vi "Load State Machine.vi"(11 "Autonomous? (Default false)":bool) -> (3 "Done (For Auto Use Only)":bool)   [LabVIEW 2013]
uses:
  typedefs/singleUseSubstate.ctl
  typedefs/fg_typedef.ctl
  typedefs/DevRef Type.ctl
  <vilib>/Rock Robotics/WPI/Solenoid/WPI_SolenoidValue.ctl
  typedefs/subStates.ctl
  <vilib>/Rock Robotics/WPI/Solenoid/WPI_SolenoidGetEnum.vi
panel:
  # "A State Machine to Handle Loading for Either High or Low Goal Shots"
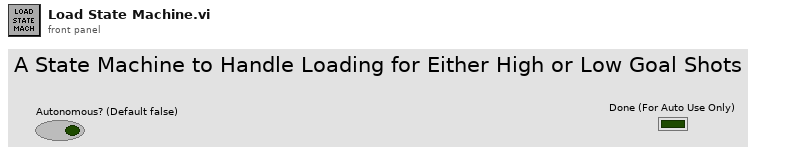
[diagram p1: front panel]
types:
  T1 = typedef "WPI_SolenoidValue.ctl" = enum16{"Off", "On", "Forward", "Reverse"}
  T2 = typedef "DevRef Type.ctl" = enum16{"Shooter Solenoid", "Latch Solenoid", "Right Up Sensor", "Right Down Sensor", "Hold Sensor", "Arm Encoder"}
  T3 = typedef "fg_typedef.ctl" = enum16{"Get", "Set"}
  T4 = typedef "singleUseSubstate.ctl" = enum16{"null", "wait", "shift high", "shift low", "extend shooter", "retract shooter", "latch", "unlatch"}
  T5 = typedef "subStates.ctl" = enum16{"null", "wait", "driver control", "auto", "manual override", "hold position", "rotate", "pickup", "pass", "load", "goto shoot", "shoot high goal", "shoot low goal", "cancel arm", "cancel shooter", "end"}
  T6 = typedef "WPI_SolenoidDevRef.ctl" = cluster{"DevStatus":errorcluster, "Solenoid Module":T7, "Forward Solenoid Channel":T8, "Reverse Solenoid Channel":T8}
  T7 = typedef "FPGA_TypedefSolenoidModule.ctl" = enum16{"Solenoid Module 1", "Solenoid Module 2"}
  T8 = typedef "WPI_SolenoidChannel.ctl" = enum8{"Solenoid 1", "Solenoid 2", "Solenoid 3", "Solenoid 4", "Solenoid 5", "Solenoid 6", "Solenoid 7", "Solenoid 8", "Invalid"}
  T9 = typedef "WPI_DigitalInputDevRef.ctl" = cluster{"DevStatus":errorcluster, "DIO Channel":T10, "Digital Module":T11}
  T10 = typedef "FPGA_DIOChannel.ctl" = enum8{"DIO 1", "DIO 2", "DIO 3", "DIO 4", "DIO 5", "DIO 6", "DIO 7", "DIO 8", "DIO 9", "DIO 10", "DIO 11", "DIO 12", "DIO 13", "DIO 14", "Invalid"}
  T11 = typedef "FPGA_TypedefDigitalModule.ctl" = enum16{"Digital Module 1", "Digital Module 2"}
  T12 = typedef "WPI_EncoderDevRef.ctl" = cluster{"DevStatus":errorcluster, "EncoderIndex":T13, "CounterIndex":T14, "DistancePerCount":dbl, "Decoding Type":T15}
  T13 = typedef "FPGA_EncoderIdx.ctl" = enum8{"Enc 0", "Enc 1", "Enc 2", "Enc 3", "Invalid"}
  T14 = typedef "FPGA_CounterCtrSystemIndex.ctl" = enum8{"Ctr 0", "Ctr 1", "Ctr 2", "Ctr 3", "Ctr 4", "Ctr 5", "Ctr 6", "Ctr 7", "Invalid"}
  T15 = typedef "WPI_EncoderType.ctl" = enum16{"1x", "2x", "4x"}
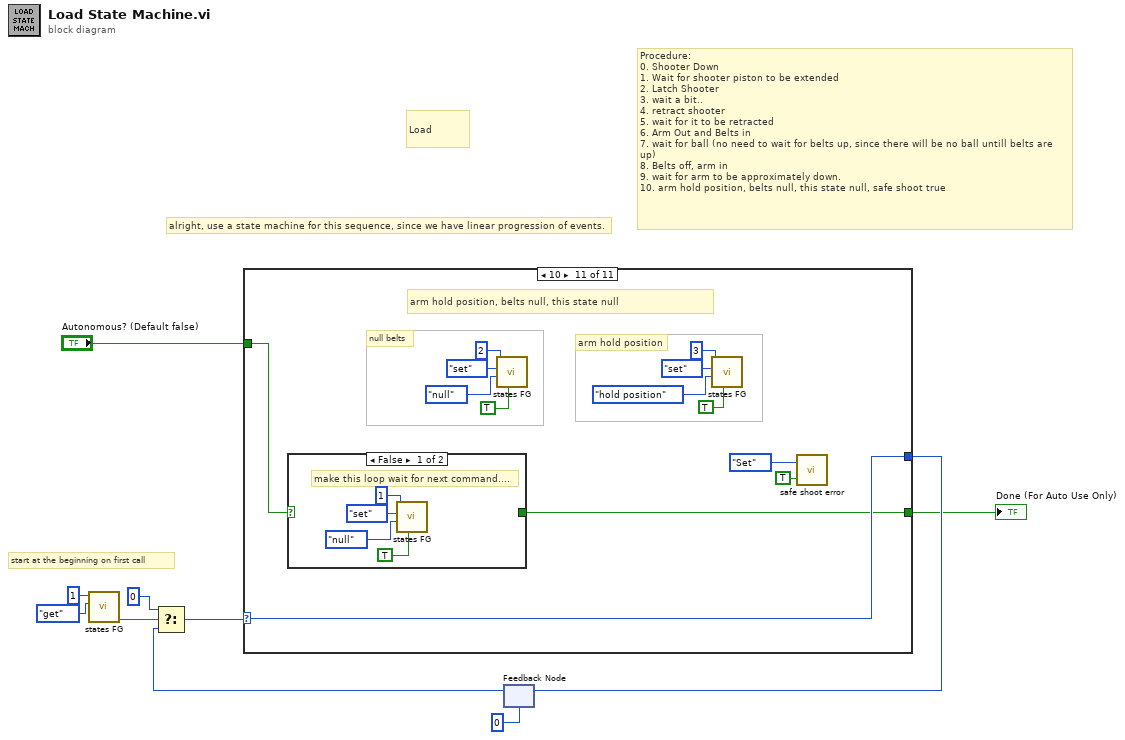
[diagram p0: block diagram]
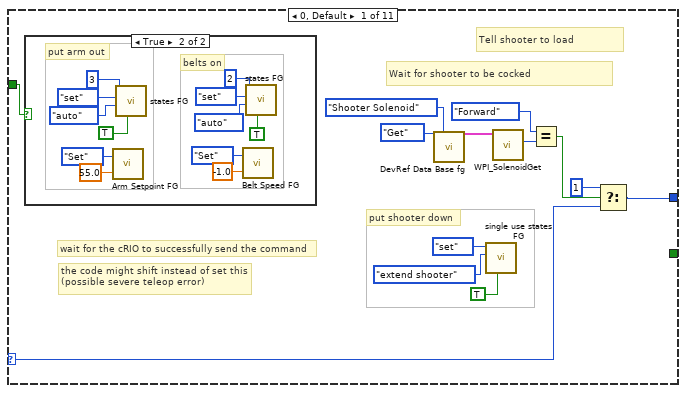
[diagram p2: hidden frame]
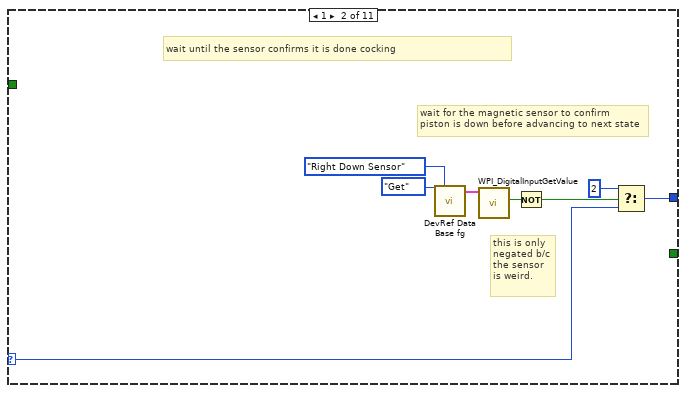
[diagram p4: hidden frame]
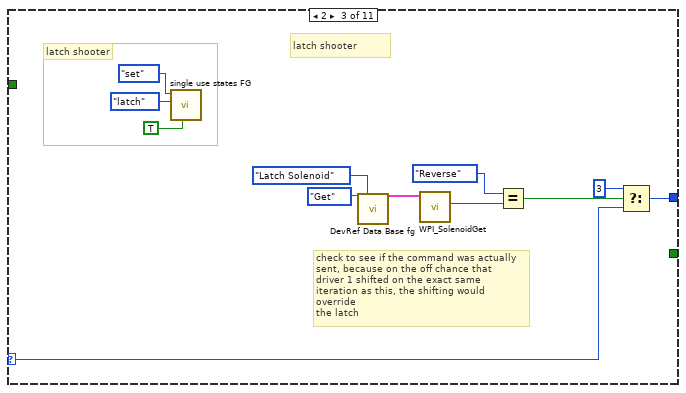
[diagram p5: hidden frame]
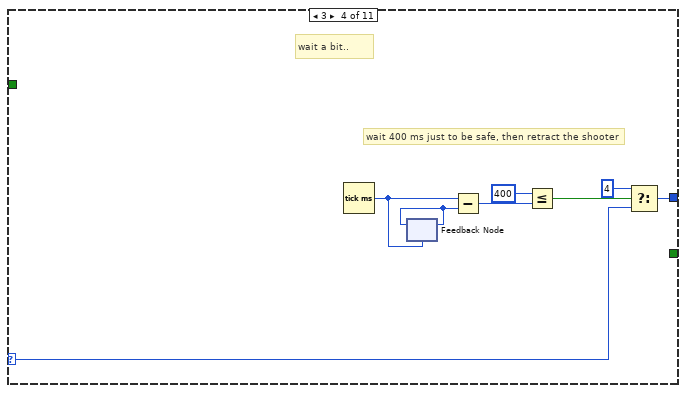
[diagram p6: hidden frame]
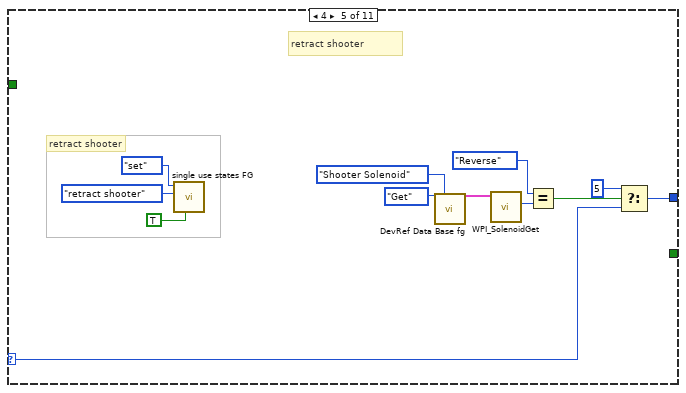
[diagram p7: hidden frame]
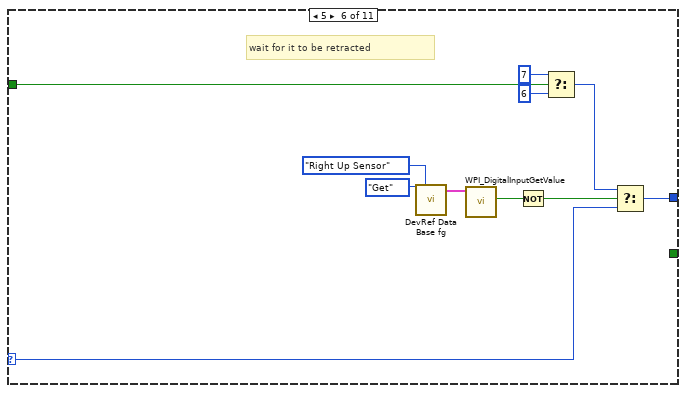
[diagram p8: hidden frame]
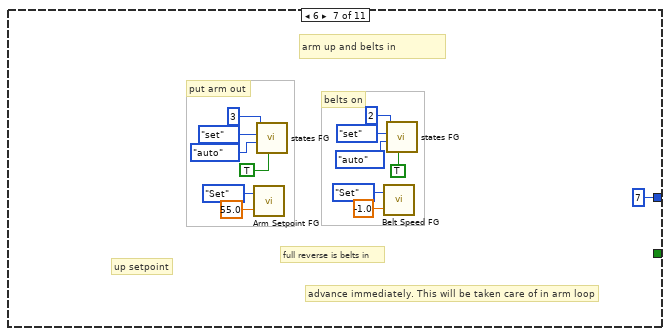
[diagram p9: hidden frame]
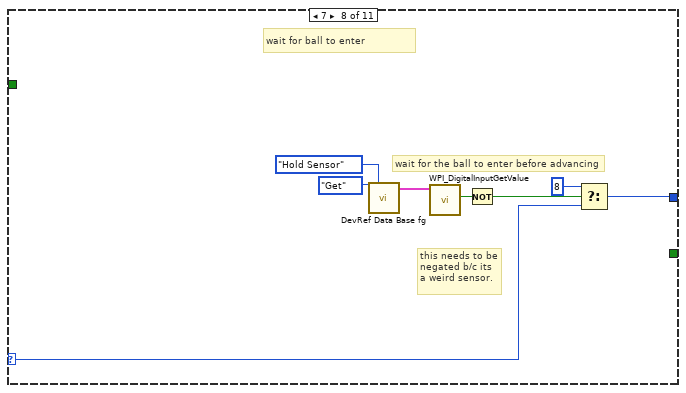
[diagram p10: hidden frame]
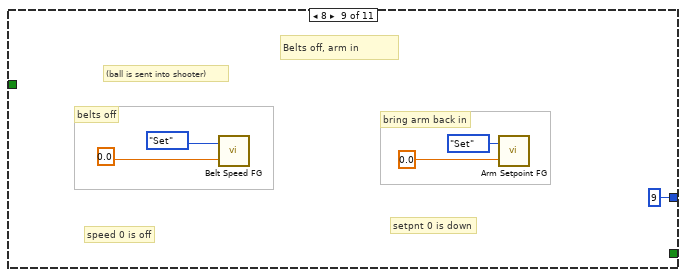
[diagram p11: hidden frame]
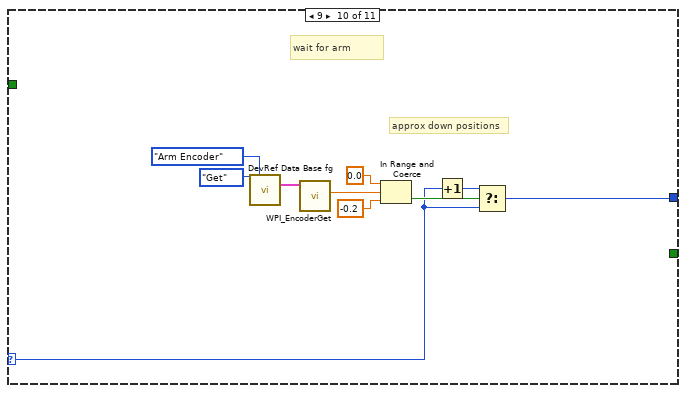
[diagram p12: hidden frame]
diagram:
  # "start at the beginning on first call"
  # "Load"
  # "Procedure: \n0. Shooter Down \n1. Wait for shooter piston to be extended\n2. Latch Shooter\n3. wait a bit..\n4. retract shooter\n5. wait for it to be retracted\n6. Arm Out and Belts in\n7. wait for ball (no need to wait for belts up, since there will be no ball untill belts are up)\n8. Belts off, arm in\n9. wait for arm to be approximately down.\n10. arm hold position, belts null, this state null, safe shoot true"
  # "alright, use a state machine for this sequence, since we have linear progression of events."
  n1 = call "states FG.vi"("menu (get)"=enum16{"set", "get"}."get", "Loop ID"=1) -> ("first call?"=w3:bool)  [unwired: 6 in, 3 out]
  n2 = feedback #1(u8 0) -> (w4:u8)
  n3 = Select(t=u8 0, s=w3, f=w4) -> (s? t:f=w6:u8)
  n4 = case shown="10" w6 {
    selector: w6 -> [w19 w38 w51 w57 w71 w81 _ w105 _ w115 w129]
    tunnel: [w20 w37 w52 w59 w70 w80 u8 7 ("t") w104 u8 9 ("t") w113 w129] -> w9
    tunnel: "Autonomous? (Default false)" -> [w11 _ _ _ _ w77 _ _ _ _ w124]
    tunnel: [_ _ _ _ _ _ _ _ _ _ w123] -> w1
    frame 0, Default {
      # "the code might shift instead of set this\n(possible severe teleop error)"
      # "Wait for shooter to be cocked"
      # "wait for the cRIO to successfully send the command"
      # "Tell shooter to load"
      # "put shooter down"
      n5 = case shown="True" w11 {
        frame False {
        }
        frame True {
          # "belts on"
          # "put arm out"
          n6 = call "Arm Setpoint FG.vi"("Setpoint In"=55.0, "Menu"=fg_typedef."Set") -> ()  [unwired: 1 out]
          n7 = call "states FG.vi"("exit in"=TRUE, "subState in"=subStates."auto", "menu (get)"=enum16{"set", "get"}."set", "Loop ID"=3) -> ()  [unwired: 4 in, 4 out]
          n8 = call "Belt Speed FG.vi"("Speed In"=-1.0 ("Setpoint In"), "Menu"=fg_typedef."Set") -> ()  [unwired: 1 out]
          n9 = call "states FG.vi"("exit in"=TRUE, "subState in"=subStates."auto", "menu (get)"=enum16{"set", "get"}."set", "Loop ID"=2) -> ()  [unwired: 4 in, 4 out]
        }
      }
      n10 = call "DevRef Data Base fg.vi"("Menu"=fg_typedef."Get", "DevRef to Get"=DevRef_Type."Shooter Solenoid") -> ("Selected Solenoid"=w16:T6)  [unwired: 23 in, 2 out]
      n11 = call "single use states FG.vi"("exit in"=TRUE, "substate"=singleUseSubstate."extend shooter", "menu (get)"=enum16{"set", "get"}."set") -> ()  [unwired: 5 in, 4 out]
      n12 = call-poly <vilib>:"WPI_SolenoidGet.vi"("SolenoidDevRef"=w16) -> ("Value"=w15:T1)  [unwired: 8 in, 2 out]
      n13 = Equal?(x=WPI_SolenoidValue."Forward", y=w15) -> (x = y?=w13:bool)
      n14 = Select(t=u8 1, s=w13, f=w19) -> (s? t:f=w20:u8)
    }
    frame 1 {
      # "this is only\nnegated b/c\nthe sensor\nis weird."
      # "wait for the magnetic sensor to confirm \npiston is down before advancing to next state"
      # "wait until the sensor confirms it is done cocking"
      n15 = call "DevRef Data Base fg.vi"("Menu"=fg_typedef."Get", "DevRef to Get"=DevRef_Type."Right Down Sensor") -> ("Selected Sensor"=w40:T9)  [unwired: 23 in, 2 out]
      n16 = call <vilib>:"WPI_DigitalInputGetValue.vi"("DigitalInputDevRef"=w40) -> ("Value"=w43:bool)  [unwired: 8 in, 2 out]
      n17 = Not(x=w43) -> (.not. x?=w42:bool)
      n18 = Select(t=u8 2, s=w42, f=w38) -> (s? t:f=w37:u8)
    }
    frame 2 {
      # "latch shooter"
      # "check to see if the command was actually\nsent, because on the off chance that\ndriver 1 shifted on the exact same\niteration as this, the shifting would override\nthe latch"
      # "latch shooter"
      n19 = call "single use states FG.vi"("exit in"=TRUE, "substate"=singleUseSubstate."latch", "menu (get)"=enum16{"set", "get"}."set") -> ()  [unwired: 5 in, 4 out]
      n20 = call "DevRef Data Base fg.vi"("Menu"=fg_typedef."Get", "DevRef to Get"=DevRef_Type."Latch Solenoid") -> ("Selected Solenoid"=w49:T6)  [unwired: 23 in, 2 out]
      n21 = call-poly <vilib>:"WPI_SolenoidGet.vi"("SolenoidDevRef"=w49) -> ("Value"=w48:T1)  [unwired: 8 in, 2 out]
      n22 = Equal?(x=WPI_SolenoidValue."Reverse" ("Value"), y=w48) -> (x = y?=w46:bool)
      n23 = Select(t=u8 3, s=w46, f=w51) -> (s? t:f=w52:u8)
    }
    frame 3 {
      # "wait a bit.."
      # "wait 400 ms just to be safe, then retract the shooter"
      n24 = Tick Count (ms)() -> (millisecond timer value=w61:u32)
      n25 = feedback #2(w61) -> (w62:u32)
      n26 = feedback-in #2(w62) -> ()
      n27 = Subtract(x=w61, y=w62) -> (x-y=w60:u32)
      n28 = Less Or Equal?(x=u32 400, y=w60) -> (x <= y?=w58:bool)
      n29 = Select(t=u8 4, s=w58, f=w57) -> (s? t:f=w59:u8)
    }
    frame 4 {
      # "retract shooter"
      # "retract shooter"
      n30 = call "single use states FG.vi"("exit in"=TRUE, "substate"=singleUseSubstate."retract shooter", "menu (get)"=enum16{"set", "get"}."set") -> ()  [unwired: 5 in, 4 out]
      n31 = call "DevRef Data Base fg.vi"("Menu"=fg_typedef."Get", "DevRef to Get"=DevRef_Type."Shooter Solenoid") -> ("Selected Solenoid"=w68:T6)  [unwired: 23 in, 2 out]
      n32 = call-poly <vilib>:"WPI_SolenoidGet.vi"("SolenoidDevRef"=w68) -> ("Value"=w67:T1)  [unwired: 8 in, 2 out]
      n33 = Equal?(x=WPI_SolenoidValue."Reverse", y=w67) -> (x = y?=w65:bool)
      n34 = Select(t=u8 5, s=w65, f=w71) -> (s? t:f=w70:u8)
    }
    frame 5 {
      # "wait for it to be retracted"
      n35 = call "DevRef Data Base fg.vi"("Menu"=fg_typedef."Get", "DevRef to Get"=DevRef_Type."Right Up Sensor") -> ("Selected Sensor"=w85:T9)  [unwired: 23 in, 2 out]
      n36 = call <vilib>:"WPI_DigitalInputGetValue.vi"("DigitalInputDevRef"=w85) -> ("Value"=w84:bool)  [unwired: 8 in, 2 out]
      n37 = Not(x=w84) -> (.not. x?=w83:bool)
      n38 = Select(t=u8 7, s=w77, f=u8 6 ("t")) -> (s? t:f=w78:u8)
      n39 = Select(t=w78, s=w83, f=w81) -> (s? t:f=w80:u8)
    }
    frame 6 {
      # "full reverse is belts in"
      # "belts on"
      # "up setpoint"
      # "arm up and belts in"
      # "advance immediately. This will be taken care of in arm loop"
      # "put arm out"
      n40 = call "Arm Setpoint FG.vi"("Setpoint In"=55.0, "Menu"=fg_typedef."Set") -> ()  [unwired: 1 out]
      n41 = call "states FG.vi"("exit in"=TRUE, "subState in"=subStates."auto", "menu (get)"=enum16{"set", "get"}."set", "Loop ID"=3) -> ()  [unwired: 4 in, 4 out]
      n42 = call "Belt Speed FG.vi"("Speed In"=-1.0 ("Setpoint In"), "Menu"=fg_typedef."Set") -> ()  [unwired: 1 out]
      n43 = call "states FG.vi"("exit in"=TRUE, "subState in"=subStates."auto", "menu (get)"=enum16{"set", "get"}."set", "Loop ID"=2) -> ()  [unwired: 4 in, 4 out]
    }
    frame 7 {
      # "this needs to be\nnegated b/c its\na weird sensor."
      # "wait for the ball to enter before advancing"
      # "wait for ball to enter"
      n44 = call "DevRef Data Base fg.vi"("Menu"=fg_typedef."Get", "DevRef to Get"=DevRef_Type."Hold Sensor") -> ("Selected Sensor"=w102:T9)  [unwired: 23 in, 2 out]
      n45 = call <vilib>:"WPI_DigitalInputGetValue.vi"("DigitalInputDevRef"=w102) -> ("Value"=w107:bool)  [unwired: 8 in, 2 out]
      n46 = Not(x=w107) -> (.not. x?=w106:bool)
      n47 = Select(t=u8 8, s=w106, f=w105) -> (s? t:f=w104:u8)
    }
    frame 8 {
      # "bring arm back in"
      # "setpnt 0 is down"
      # "speed 0 is off"
      # "Belts off, arm in"
      # "(ball is sent into shooter)"
      # "belts off"
      n48 = call "Belt Speed FG.vi"("Speed In"=0.0 ("Setpoint In"), "Menu"=fg_typedef."Set") -> ()  [unwired: 1 out]
      n49 = call "Arm Setpoint FG.vi"("Setpoint In"=0.0, "Menu"=fg_typedef."Set") -> ()  [unwired: 1 out]
    }
    frame 9 {
      # "approx down positions"
      # "wait for arm"
      n50 = call "DevRef Data Base fg.vi"("Menu"=fg_typedef."Get", "DevRef to Get"=DevRef_Type."Arm Encoder") -> ("Selected Encoder"=w120:T12)  [unwired: 23 in, 2 out]
      n51 = call <vilib>:"WPI_EncoderGet.vi"("EncoderDevRef"=w120) -> ("Distance"=w119:dbl)  [unwired: 5 in, 5 out]
      n52 = In Range and Coerce(upper limit=0.0, x=w119, lower limit=-0.2) -> (In Range?=w116:bool)  [unwired: 1 out]
      n53 = Increment(x=w115) -> (x+1=w114:u8)
      n54 = Select(t=w114, s=w116, f=w115) -> (s? t:f=w113:u8)
    }
    frame 10 {
      # "arm hold position, belts null, this state null"
      # "arm hold position"
      # "null belts"
      n55 = case shown="False" w124 {
        selector: w124 -> [_ w140]
        tunnel: [_ w140] -> w123
        frame False {
          # "make this loop wait for next command...."
          n56 = call "states FG.vi"("exit in"=TRUE, "subState in"=subStates."null", "menu (get)"=enum16{"set", "get"}."set", "Loop ID"=1) -> ()  [unwired: 4 in, 4 out]
        }
        frame True {
        }
      }
      n57 = call "states FG.vi"("exit in"=TRUE, "subState in"=subStates."null", "menu (get)"=enum16{"set", "get"}."set", "Loop ID"=2) -> ()  [unwired: 4 in, 4 out]
      n58 = call "states FG.vi"("exit in"=TRUE, "subState in"=subStates."hold position", "menu (get)"=enum16{"set", "get"}."set", "Loop ID"=3) -> ()  [unwired: 4 in, 4 out]
      n59 = call "safe shoot error.vi"("Can Shoot Safely?"=TRUE, "Menu"=fg_typedef."Set") -> ()  [unwired: 1 out]
    }
  }
  "Done (For Auto Use Only)" <- w1
  n60 = feedback-in #1(w9) -> ()
